vi "Filter Messages.vi"(6 "Mode":u8(ring) items=["Msg Standard 11bit ID"=0, "Msg Extended 29bit ID"=2], 8 "error in":errorcluster, 9 "To ID":u32, 10 "From ID":u32, 11 "TPCANHandle in":T2=81 items=["PCAN_NONEBUS"=0, "PCAN_USBBUS1"=81, "PCAN_USBBUS2"=82, "PCAN_USBBUS3"=83, "PCAN_USBBUS4"=84, "PCAN_USBBUS5"=85, "PCAN_USBBUS6"=86, "PCAN_USBBUS7"=87, "PCAN_USBBUS8"=88, "PCAN_USBBUS9"=1289, "PCAN_USBBUS10"=1290, "PCAN_USBBUS11"=1291, "PCAN_USBBUS12"=1292, "PCAN_USBBUS13"=1293, "PCAN_USBBUS14"=1294, "PCAN_USBBUS15"=1295, "PCAN_USBBUS16"=1296]) -> (0 "error out":errorcluster, 3 "TPCANHandle out":T2=81 items=["PCAN_NONEBUS"=0, "PCAN_USBBUS1"=81, "PCAN_USBBUS2"=82, "PCAN_USBBUS3"=83, "PCAN_USBBUS4"=84, "PCAN_USBBUS5"=85, "PCAN_USBBUS6"=86, "PCAN_USBBUS7"=87, "PCAN_USBBUS8"=88, "PCAN_USBBUS9"=1289, "PCAN_USBBUS10"=1290, "PCAN_USBBUS11"=1291, "PCAN_USBBUS12"=1292, "PCAN_USBBUS13"=1293, "PCAN_USBBUS14"=1294, "PCAN_USBBUS15"=1295, "PCAN_USBBUS16"=1296], 5 "TPCANStatus":T1 items=["PCAN_ERROR_OK"=0, "PCAN_ERROR_XMTFULL"=1, "PCAN_ERROR_OVERRUN"=2, "PCAN_ERROR_BUSLIGHT"=4, "PCAN_ERROR_BUSHEAVY"=8, "PCAN_ERROR_BUSPASSIVE"=262144, "PCAN_ERROR_BUSOFF"=16, "PCAN_ERROR_QRCVEMPTY"=32, "PCAN_ERROR_QOVERRUN"=64, "PCAN_ERROR_QXMTFULL"=128, "PCAN_ERROR_REGTEST"=256, "PCAN_ERROR_NODRIVER"=512, "PCAN_ERROR_HWINUSE"=1024, "PCAN_ERROR_NETINUSE"=2048, "PCAN_ERROR_ILLHW"=5120, "PCAN_ERROR_ILLNET"=6144, "PCAN_ERROR_ILLCLIENT"=7168, "PCAN_ERROR_RESOURCE"=8192, "PCAN_ERROR_ILLPARAMTYPE"=16384, "PCAN_ERROR_ILLPARAMVAL"=32768, "PCAN_ERROR_UNKNOWN"=65536, "PCAN_ERROR_ILLDATA"=131072, "PCAN_ERROR_ILLMODE"=524288, "PCAN_ERROR_CAUTION"=33554432, "PCAN_ERROR_INITIALIZE"=67108864, "PCAN_ERROR_ILLOPERATION"=134217728])   [LabVIEW 2019, in "PCANBasic.lvlib"]
doc: "Configures the reception filter.\n\nNote that after a PCAN Channel is initialized, the status of its filter is fully opened. According with the current filter status, calling this function causes the following behavior:\n\nFilter status is PCAN_FILTER_OPEN: The filter is automatically closed and then configured with the given range of IDs passed to this function [FromID, ToID] . \nFilter status is PCAN_FILTER_CLOSE: The filter is set to the given range of IDs passed to this function [FromID, ToID] . \nFilter status is PCAN_FILTER_CUSTOM: The filter is expanded with the given range of Ids [FromID, ToID]. If a smaller or different range is required than a range that has been configured before, the filter has to be closed first before calling the CAN_FilterMessages function. To do this use the function CAN_SetValue. \nThe parameter 'Mode' indicates which kind of ID is being used to register the new filter range. There are two possible values, Standard (11-bit identifier) or Extended (29-bit identifier). Standard frames are using the bit positions 28 to 18 of the Acceptance Mask/Code registers in the SJA1000 CAN controller. Drivers for 82C200 CAN controllers have to shift the bits down to positions 10 to 0. \n\nTake in account that configuring the message filter cause the CAN controller to enter the reset state. This will affect other applications that communicate with the same PCAN hardware. \n\nNotes: \n\nThere is only one filter for standard and extended CAN messages. It seems that the ID from a standard message uses the most significant 11 bits (bit 18 to 28) of the 29 bits. I.e. the standard ID 400h is also received by indicating an extended ID 10000000h. For this reason, it is not recommended to mix standard and extended filters, since it can increase the risk of receiving unwanted messages. \nMultiple calls of CAN_FilterMessages expand the reception filter. \nIt is not guaranteed that an application only receives CAN messages in the range of FromID to ToID. This is caused by the operating principle of the SJA1000's acceptance filter. See also Philips Data Sheet \"SJA1000 Stand-alone CAN-controller\"."
uses:
  PCANBasic.lvlib
  TPCANHandle.ctl
  TPCANStatus.ctl
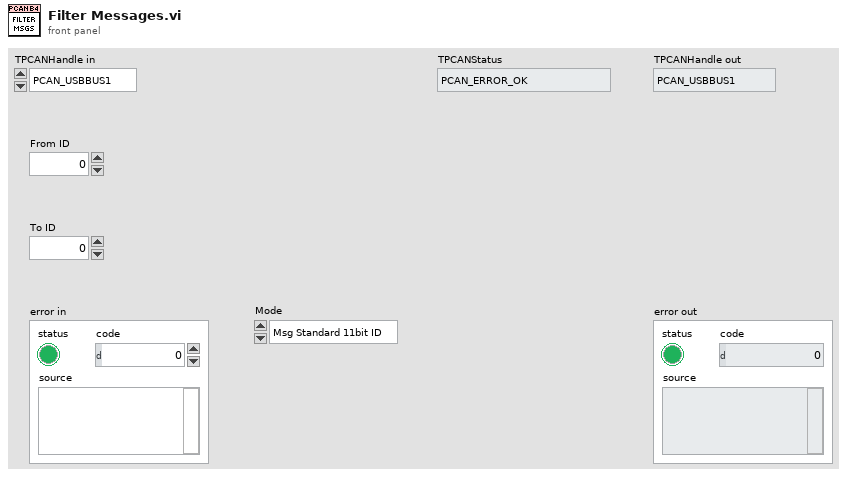
[diagram p1: front panel]
types:
  T1 = typedef "PCANBasic.lvlib/TPCANStatus.ctl" = u32
  T2 = typedef "PCANBasic.lvlib/TPCANHandle.ctl" = u16
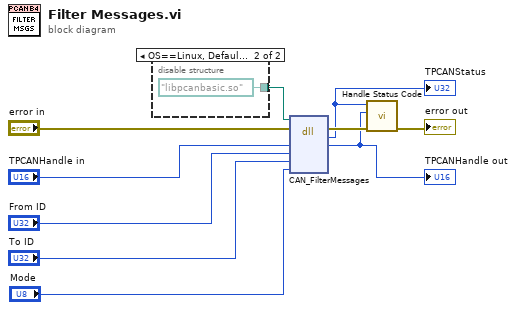
[diagram p0: block diagram]
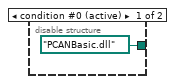
[diagram p2: hidden frame]
diagram:
  n1 = disable-structure shown="OS==Linux, Default" {
    disable-tunnel: [path "PCANBasic.dll" path "libpcanbasic.so"] -> w10
    frame condition #0 (active) {
    }
    frame condition #1 {
    }
  }
  n2 = dll-call lib="?" fn="CAN_FilterMessages"(path in=w10, error in="error in", "Channel"="TPCANHandle in", "FromID"="From ID", "ToID"="To ID", "Mode"="Mode") -> (error out=w7:errorcluster, "TPCANStatus"=w5:u32, "Channel"=w1:u16)  [unwired: 4 in, 1 out]
  "TPCANHandle out" <- w1
  "TPCANStatus" <- w5
  n3 = call "Handle Status Code.vi"("error in"=w7, "TPCANHandle"=w1, "TPCANStatus"=w5) -> ("error out"=→"error out":errorcluster)  [unwired: 8 in]
